vi "2D to 1D Array.vi"(10 "2D array":dbl[][](array[numeric])) -> (2 "1D Array":dbl[](array[numeric]))   [LabVIEW 2016]
panel:
  out "size(s)":i32[](array[numeric])
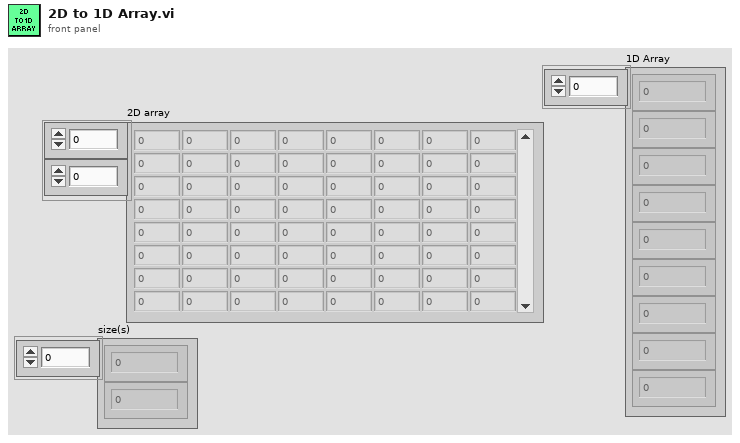
[diagram p1: front panel]
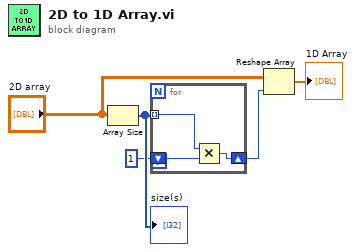
[diagram p0: block diagram]
diagram:
  n1 = Array Size(array="2D array") -> (size(s)=w3:i32[])
  "size(s)" <- w3
  n2 = for {
    tunnel: w3 -> [w8] mode=indexing
    shift-right: [w6] -> w1
    shift-left: 1 ("dimension size") -> [w7]
    n3 = Multiply(x=w8, y=w7) -> (x*y=w6:i32)
  }
  n4 = Reshape Array("2D array", w1) -> (→"1D Array":dbl[])
